vi "printDirectory.vi"(8 "Error In":errorcluster, 10 "nested level":u8, 11 "file":refnum<class "File.lvclass">) -> (0 "Error Out":errorcluster)   [LabVIEW 2014]
uses:
  LabVIEW-Universal-Transcriptor-SD-Card-Library/File.lvclass
  LabVIEW-Universal-Transcriptor-SD-Card-Library/File.lvclass/File.ctl
  LabVIEW-Universal-Transcriptor-SD-Card-Library/File Class/Get If Rewind This Directory.vi
  <vilib>/Utility/file.llb/Application Directory.vi
  LabVIEW-Universal-Transcriptor-SD-Card-Library/open.vi
  <vilib>/LabVIEW Universal Transcriptor/LabVIEW to Arduino Transcriptor/Transcriptors/System API/Serial println string.vi
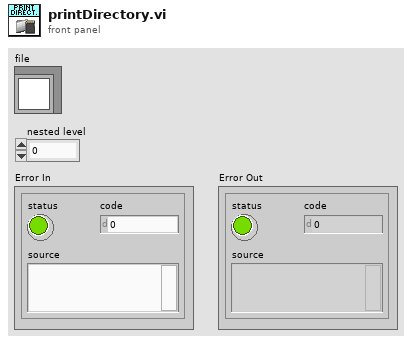
[diagram p1: front panel]
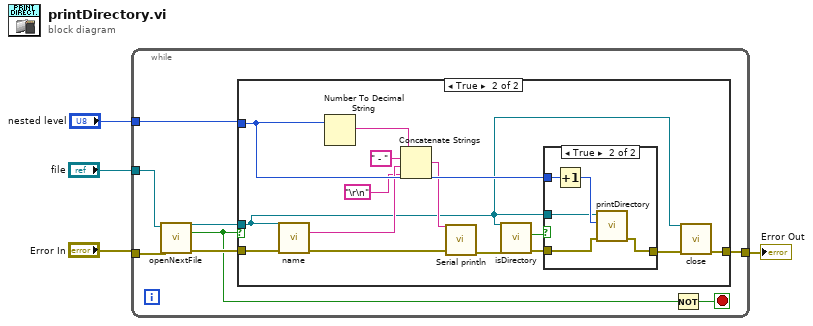
[diagram p0: block diagram]
diagram:
  n1 = while {
    tunnel: "nested level" -> [w9]
    tunnel: "Error In" -> [w6]
    tunnel: [w10] -> w3
    tunnel: "file" -> [w5]
    stop <- w8 stop-if-true
    n2 = call "openNextFile.vi"("error in (no error)"=w6, "File in"=w5) -> ("error out"=w11:errorcluster, "success?"=w7:bool, "File out"=w12:refnum<class "File.lvclass">)  [unwired: 7 in]
    n3 = case shown="True" w7 {
      tunnel: w12 -> [_ w16]
      tunnel: w11 -> [w13 w27]
      tunnel: [w13 w18] -> w10
      tunnel: w9 -> [_ w23]
      frame False {
      }
      frame True {
        n4 = call-dynamic "name.vi"("error in (no error)"=w27, "File in"=w16) -> ("error out"=w26:errorcluster, "file name"=w17:string)  [unwired: 8 in]
        n5 = Number To Decimal String(number=w23) -> (decimal integer string=w22:string)  [unwired: 1 in]
        n6 = Concatenate Strings(w22, " - " ("string"), w17, "\r\n") -> (w20:string)
        n7 = call-poly <vilib>:"Serial println.vi"("Error In"=w26, "string in"=w20) -> ("Error Out"=w25:errorcluster)  [unwired: 9 in]
        n8 = call-dynamic "isDirectory.vi"("error in (no error)"=w25, "File in"=w16) -> ("error out"=w24:errorcluster, "is directory?"=w15:bool)  [unwired: 8 in]
        n9 = case shown="True" w15 {
          tunnel: w24 -> [w28 w32]
          tunnel: [w28 w31] -> w19
          tunnel: w16 -> [_ w29]
          tunnel: w23 -> [_ w33]
          frame False {
          }
          frame True {
            n10 = Increment(x=w33) -> (x+1=w30:u8)
            n11 = call "printDirectory.vi"("Error In"=w32, "nested level"=w30, "file"=w29) -> ("Error Out"=w31:errorcluster)  [unwired: 8 in]
          }
        }
        n12 = call-dynamic "close.vi"("error in (no error)"=w19, "File in"=w16) -> ("error out"=w18:errorcluster)  [unwired: 9 in]
      }
    }
    n13 = Not(x=w7) -> (.not. x?=w8:bool)
  }
  "Error Out" <- w3
